vi "Correct Taus.vi"(4 "#_shots":i32=5, 6 "Filter?":bool, 8 "error in":errorcluster, 9 "filter changed?":bool, 11 "CRDS Cell in":refnum<class "CRDS Cell.lvclass">) -> (0 "error out":errorcluster, 3 "CRDS Cell out":refnum<class "CRDS Cell.lvclass">)   [LabVIEW 2019, in "CRDS Cell.lvclass"]
doc: "Correct tau values for Rayleigh scattering. \n\nIf on filter:\n* The tau and tau0 values will be the uncorrected values in seconds.\n* tau0corr will be in the Rayleigh scattering corrected value in us.\n* ext, extcorr and taucorr will be set to NaN.\n\nIf on sample:\n* Tau is the raw tau value in us.\n* taucorr will be the Rayleigh scattering corrected value in us\n* ext and extCorr will be the same value."
uses:
  CRDS Cell.lvclass
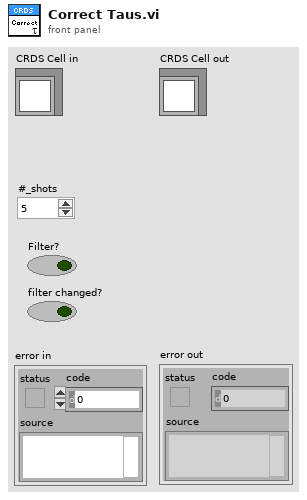
[diagram p1: front panel]
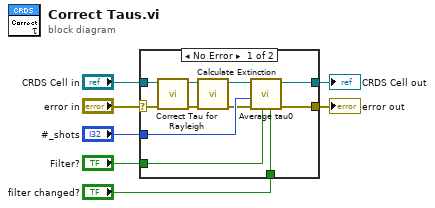
[diagram p0: block diagram]
diagram:
  n1 = case shown="No Error" "error in" {
    selector: "error in" -> [w9 w20]
    tunnel: [w17 w20] -> w3
    tunnel: [w18 w19] -> w2
    tunnel: "CRDS Cell in" -> [w11 w19]
    tunnel: "Filter?" -> [w14 _]
    tunnel: "#_shots" -> [w16 _]
    tunnel: "filter changed?" -> [w15 _]
    frame No Error {
      n2 = call "Correct Tau for Rayleigh.vi"("error in (no error)"=w9, "CRDS Cell in"=w11) -> ("error out"=w13:errorcluster, "CRDS Cell Out"=w12:refnum<class "CRDS Cell.lvclass">)  [unwired: 8 in]
      n3 = call "Calculate Extinction.vi"("error in"=w13, "CRDS Cell in"=w12) -> ("error out"=w8:errorcluster, "CRDS Cell out"=w10:refnum<class "CRDS Cell.lvclass">)  [unwired: 8 in]
      n4 = call "Average tau0.vi"("filter changed?"=w15, "filter"=w14, "error in"=w8, "# of shots"=w16, "CRDS Cell in"=w10) -> ("error out"=w17:errorcluster, "CRDS Cell out"=w18:refnum<class "CRDS Cell.lvclass">)  [unwired: 5 in]
    }
    frame Error {
    }
  }
  "error out" <- w3
  "CRDS Cell out" <- w2
